vi "uTTA_GetCAL_Output.vi"(6 "Number of Samples":u32=10, 8 "error in":errorcluster, 9 "Timeout(ms)":i32=5000, 10 "RX Termination(\\n)":string="\n", 11 "VISA Refnum in":refnum<visa-resource-name>) -> (0 "error out":errorcluster, 1 "Temperatures":dbl[][](array[numeric]), 2 "ADCs":i32[][](array[numeric]), 3 "VISA Refnum out":refnum<visa-resource-name>, 4 "PGA":i32[](array[numeric]))   [LabVIEW 2021]
panel:
  out "Timeout":bool
  out "Received":string
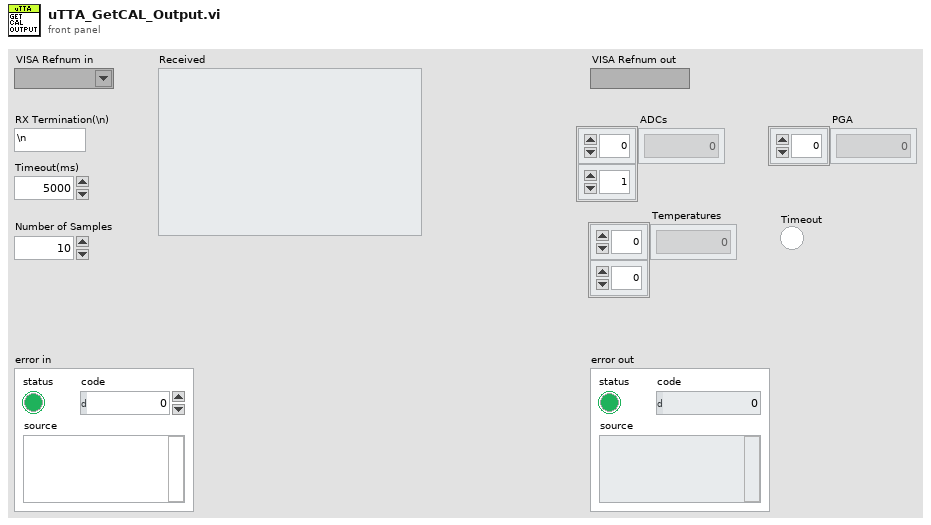
[diagram p1: front panel]
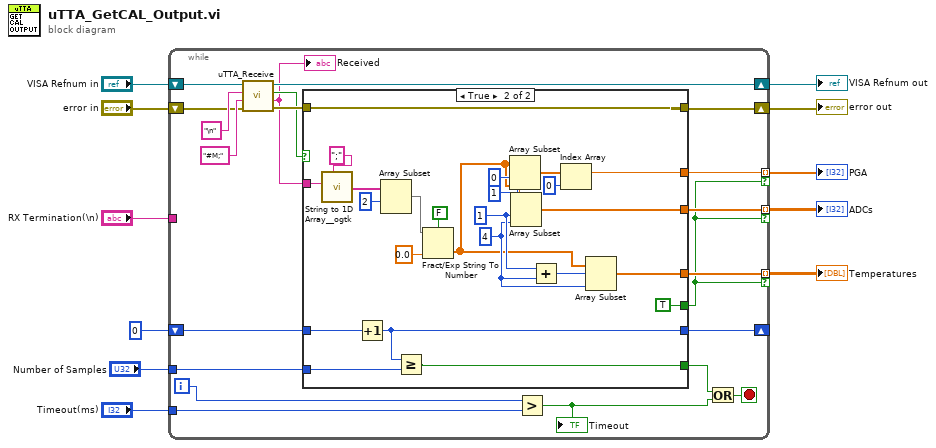
[diagram p0: block diagram]
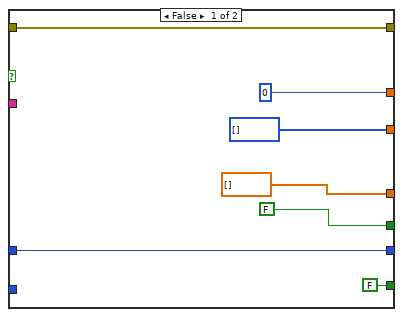
[diagram p2: hidden frame]
diagram:
  n1 = while {
    tunnel: "RX Termination(\\n)" -> [_]
    tunnel: "Timeout(ms)" -> [w18]
    tunnel: [w32] -> w5 mode=indexing if=w29
    tunnel: [w31] -> w4 mode=indexing if=w29
    shift-right: [w30] -> w8
    shift-left: "error in" -> [w24]
    shift-right: [w23] -> w9
    shift-left: "VISA Refnum in" -> [w25]
    tunnel: [w28] -> w3 mode=indexing if=w29
    tunnel: "Number of Samples" -> [w17]
    shift-right: [w15] -> _
    shift-left: 0 ("Timeout(ms)") -> [w16]
    i -> [w19]
    stop <- w12 stop-if-true
    n2 = call "uTTA_Receive.vi"("error in (no error)"=w24, "Response Qualifier(\"\")"="#M;" ("Response Qualifier(\"\")"), "RX Termination(\\n)"="\n" ("RX Termination(\\n)"), "VISA Refnum in"=w25) -> ("error out"=w22:errorcluster, "Response"=w20:string, "Found response"=w21:bool, "VISA Refnum out"=w23:refnum<visa-resource-name>)  [unwired: 4 in]
    "Received" <- w20
    n3 = case shown="True" w21 {
      tunnel: [i32[] [] w61] -> w32
      tunnel: [dbl[] [] w40] -> w31
      tunnel: w22 -> [w38 w63]
      tunnel: [w38 w63] -> w30
      tunnel: [FALSE TRUE] -> w29
      tunnel: [0 w54] -> w28
      tunnel: w20 -> [_ w46]
      tunnel: w17 -> [_ w44]
      tunnel: w16 -> [w34 w45]
      tunnel: [FALSE w43] -> w14
      tunnel: [w34 w42] -> w15
      frame False {
      }
      frame True {
        w58 = 4 ("length")
        w60 = 1 ("index")
        n4 = call <userlib>:"String to 1D Array__ogtk.vi"("delimiter (Tab)"=";", "string"=w46) -> ("Array of Strings"=w50:string[])  [unwired: 9 in]
        n5 = Increment(x=w45) -> (x+1=w42:i32)
        n6 = Array Subset(array=w50, index=2) -> (w47:string[])  [unwired: 1 in]
        n7 = Greater Or Equal?(x=w42, y=w44) -> (x >= y?=w43:bool)
        n8 = Fract/Exp String To Number(use system decimal point (T)=FALSE, string=w47, default (0 dbl)=0.0 ("default (0 I32)")) -> (number=w51:dbl[])  [unwired: 1 in, 1 out]
        n9 = Array Subset(array=w51, index=0, length=1) -> (w55:dbl[])
        n10 = Array Subset(array=w51, index=w60, length=w58) -> (w61:dbl[])
        n11 = Add(x=w60, y=w58) -> (x+y=w59:i32)
        n12 = Index Array(array=w55, index=0) -> (element=w54:dbl)
        n13 = Array Subset(array=w51, index=w59, length=w58) -> (w40:dbl[])
      }
    }
    n14 = Greater?(x=w19, y=w18) -> (0:w13:bool)
    "Timeout" <- w13
    n15 = Or(x=w14, y=w13) -> (x .or. y?=w12:bool)
  }
  "VISA Refnum out" <- w9
  "error out" <- w8
  "ADCs" <- w5
  "Temperatures" <- w4
  "PGA" <- w3
